vi "数值控件显示格式.vi"() -> ()   [LabVIEW 2023]
doc: "本VI是为《我和LabVIEW》一书编写的示例。\n关于本书的介绍请参考网页：\nhttp://ruanqizhen.spaces.live.com/blog/cns!5852D4F797C53FB6!4310.entry"
panel:
  in  "数值 2":i32=123456789 format="十进制：    %d\n十六进制：%08x\n二进制：    %032b"
  in  "数值":dbl format="%<%Y-%m-%d %H:%M:%S>T"
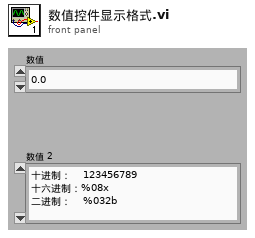
[diagram p1: front panel]
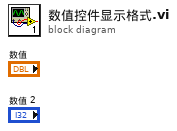
[diagram p0: block diagram]
diagram:
